vi "ID.Convert.Raw.vi"(11 "identifier":u32) -> (3 "Data":u8[](array[numeric]))   [LabVIEW 2019, in "Diagnostics Addon Engine.lvlib"]
uses:
  Diagnostics Addon Engine.lvlib
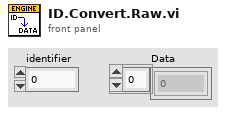
[diagram p1: front panel]
types:
  T1 = enum16{"big-endian, network order", "native, host order", "little-endian"}
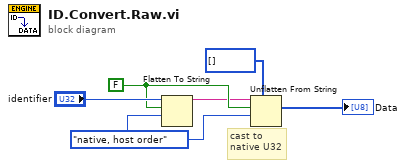
[diagram p0: block diagram]
diagram:
  w3 = FALSE ("prepend array or string size? (T)")
  w2 = T1."native, host order" ("byte order (0:big-endian, network order)")
  # "cast to \nnative U32"
  n1 = Flatten To String(anything="identifier", prepend array or string size? (T)=w3, byte order (0:big-endian, network order)=w2) -> (data string=w1:string)  [unwired: 1 in, 2 out]
  n2 = Unflatten From String(type=u8[] [], binary string=w1, data includes array or string size? (T)=w3, byte order (0:big-endian, network order)=w2) -> (value=→"Data":u8[])  [unwired: 1 in, 2 out]
